vi "load_recovery_binary.vi"(8 "error in (no error)":errorcluster, 11 "Path":path) -> (0 "error out":errorcluster, 3 "Data":dbl[](array[numeric]))   [LabVIEW 2024]
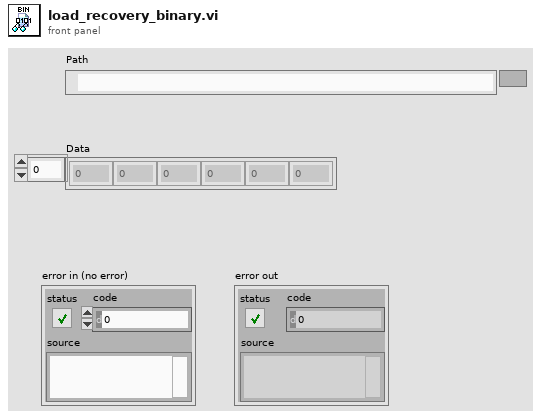
[diagram p1: front panel]
types:
  T1 = enum16{"open", "replace", "create", "open or create", "replace or create", "replace or create with confirmation"}
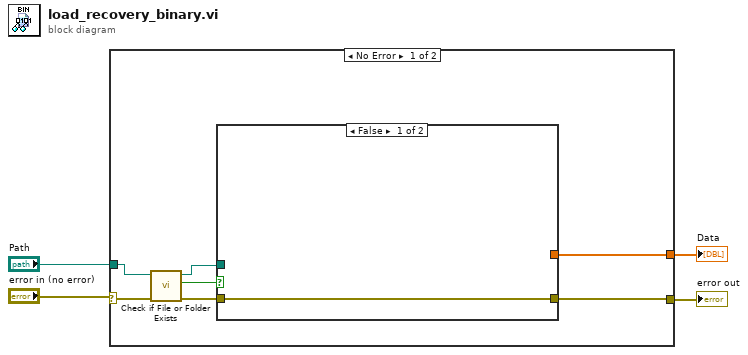
[diagram p0: block diagram]
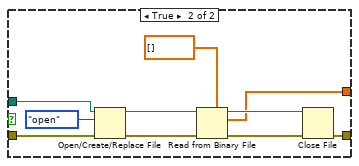
[diagram p2: hidden frame]
diagram:
  n1 = case shown="No Error" "error in (no error)" {
    selector: "error in (no error)" -> [w11 w23]
    tunnel: [w10 w23] -> w4
    tunnel: "Path" -> [w7 _]
    tunnel: [w9 _] -> w2
    frame No Error {
      n2 = call <vilib>:"Check if File or Folder Exists.vi"("error in (no error)"=w11, "path"=w7) -> ("error out"=w8:errorcluster, "file or folder exists?"=w5:bool, "dup path"=w6:path)  [unwired: 7 in]
      n3 = case shown="False" w5 {
        tunnel: w8 -> [w12 w22]
        tunnel: [w12 w19] -> w10
        tunnel: w6 -> [_ w18]
        tunnel: [_ w13] -> w9
        frame False {
        }
        frame True {
          n4 = Open/Create/Replace File(file path (use dialog)=w18, error in=w22, operation (0:open)=T1."open") -> (refnum out=w16:refnum<file>, error out=w21:errorcluster)  [unwired: 3 in, 1 out]
          n5 = Read from Binary File(5:dbl[] [], 8:w21, 11:w16) -> (0:w20:errorcluster, 2:w13:dbl[], 3:w15:refnum<file>)  [unwired: 3 in, 1 out]
          n6 = Close File(refnum=w15, error in=w20) -> (error out=w19:errorcluster)  [unwired: 1 out]
        }
      }
    }
    frame Error {
    }
  }
  "error out" <- w4
  "Data" <- w2
